vi "Configure Measurement.vi"(0 "VISA resource name":refnum<visa-resource-name>, 5 "First Channel (1: Channel A)":u16(ring)=1 items=["Channel A"=1, "Channel B"=2], 7 "Second Channel (2: Channel B)":u16(ring)=2 items=["Channel A"=1, "Channel B"=2], 9 "Measurement Function (0: Single)":u16(ring) items=["Single", "Difference", "Ratio"], 11 "error in (no error)":errorcluster) -> (4 "VISA resource name out":refnum<visa-resource-name>, 15 "error out":errorcluster)   [LabVIEW 2013, in "Template - Power Meter.lvlib"]
doc: "Configures the instrument to take single or dual channel measurements."
uses:
  <instrlib>/_Template - Power Meter/Template - Power Meter.lvlib
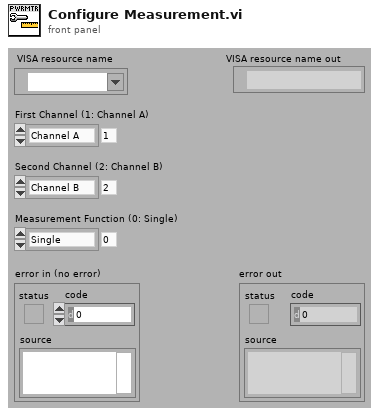
[diagram p1: front panel]
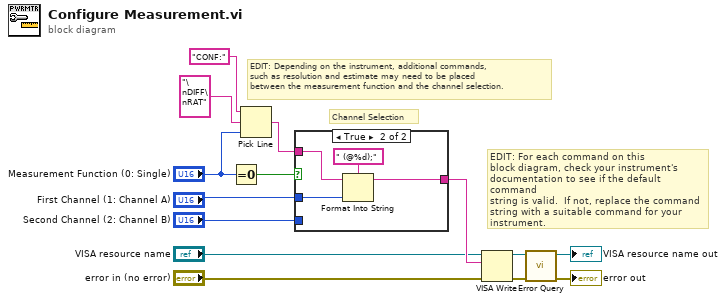
[diagram p0: block diagram]
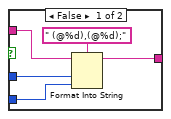
[diagram p2: hidden frame]
diagram:
  # "Channel Selection"
  # "EDIT: For each command on this\nblock diagram, check your instrument's\ndocumentation to see if the default command\nstring is valid.  If not, replace the command\nstring with a suitable command for your\ninstrument."
  # "EDIT: Depending on the instrument, additional commands, \nsuch as resolution and estimate may need to be placed\nbetween the measurement function and the channel selection."
  n1 = Equal To 0?(x="Measurement Function (0: Single)") -> (x = 0?=w9:bool)
  n2 = Pick Line(string ("")="CONF:" ("initial string"), multi-line string="\nDIFF\nRAT", line index="Measurement Function (0: Single)") -> (output string=w4:string)
  n3 = case shown="True" w9 {
    tunnel: [w19 w22] -> w14
    tunnel: "First Channel (1: Channel A)" -> [w17 w21]
    tunnel: "Second Channel (2: Channel B)" -> [w16 _]
    tunnel: w4 -> [w15 w20]
    frame False {
      n4 = Format Into String(format string=" (@%d),(@%d);", initial string=w15, w17, w16) -> (resulting string=w19:string)  [unwired: 1 in, 1 out]
    }
    frame True {
      n5 = Format Into String(format string=" (@%d);", initial string=w20, w21) -> (resulting string=w22:string)  [unwired: 1 in, 1 out]
    }
  }
  n6 = VISA Write(VISA resource name="VISA resource name", write buffer=w14, error in (no error)="error in (no error)") -> (VISA resource name out=w8:refnum<visa-resource-name>, error out=w7:errorcluster)  [unwired: 1 out]
  n7 = call <instrlib>:"Error Query.vi"("error in (no error)"=w7, "VISA resource name"=w8) -> ("error out"=→"error out":errorcluster, "VISA resource name out"=→"VISA resource name out":refnum<visa-resource-name>)  [unwired: 6 in, 2 out]
